vi "Controller - STOP ALL Actors.vi"(8 "error in":errorcluster) -> (0 "error out":errorcluster)   [LabVIEW 2023, in "Controller.lvlib" / "Controller.lvclass"]
uses:
  Controller.lvclass
  Controller - Ctrl - FGV - Action.ctl
  <vilib>/ActorFramework/Message Enqueuer/Message Enqueuer.lvclass/Message Enqueuer.ctl
  <vilib>/ActorFramework/Message Enqueuer/Enqueue.vi
  <vilib>/ActorFramework/Stop Msg/Stop Msg.lvclass
  Applications/National Instruments/LabVIEW 2023 64-bit/vi.lib/ActorFramework/Message/Message.lvclass
  <vilib>/ActorFramework/Message Priority Queue/Priority Enqueue.vi
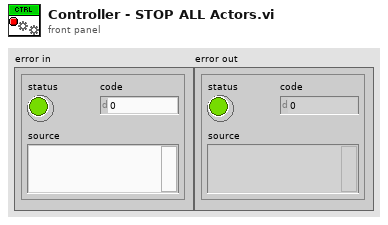
[diagram p1: front panel]
types:
  T1 = typedef "Controller.lvlib/Controller.lvclass/Controller - Ctrl - FGV - Action.ctl" = enum16{"Int", "Get"}
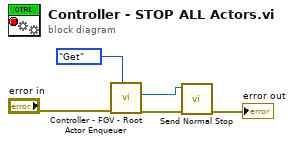
[diagram p0: block diagram]
diagram:
  n1 = call "Controller - FGV - Root Actor Enqueuer.vi"("Action"=Controller_-_Ctrl_-_FGV_-_Action."Get", "error in"="error in") -> ("error out"=w4:errorcluster, "Root Enqueuer"=w3:refnum<class "Message Enqueuer.lvclass">)  [unwired: 8 in]
  n2 = call <vilib>:"Send Normal Stop.vi"("error in (no error)"=w4, "Message Enqueuer"=w3) -> ("error out"=→"error out":errorcluster)  [unwired: 9 in]
